vi "aal_Complex Modulator(complex input).vi"(1 "reset ?":bool, 2 "fs":dbl=1024.0 min=-0.5 max=0.5 format="%.2f", 3 "frequency":dbl min=-0.5 max=0.5 format="%.2f", 4 "x":cdb[](array[numeric])) -> (0 "y":cdb[](array[numeric]))   [LabVIEW 2017, in "NI_AALPro.lvlib"]
doc: "Modulates the signal to frequency. The center frequency should be normalized (-0.5, 0.5)."
uses:
  NI_AALPro.lvlib
  <resource>/lvanlys.dll
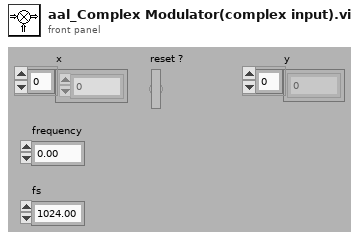
[diagram p1: front panel]
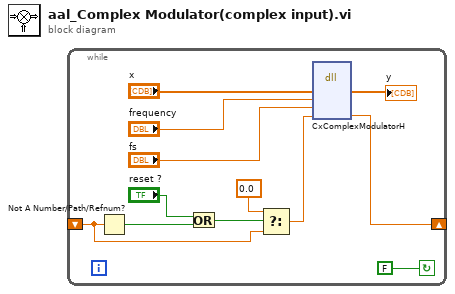
[diagram p0: block diagram]
diagram:
  n1 = while {
    shift-left: _ -> [w11]
    shift-right: [w6] -> _
    stop <- FALSE continue-if-true
    n2 = Not A Number/Path/Refnum?(number/path/refnum=w11) -> (NaN/Path/Refnum?=w2:bool)
    n3 = Or(x="reset ?", y=w2) -> (x .or. y?=w5:bool)
    n4 = Select(t=0.0, s=w5, f=w11) -> (s? t:f=w7:dbl)
    n5 = dll-call lib="C:/Program Files (x86)/National Instruments/LabVIEW 2017/resource/lvanlys.*" fn="CxComplexModulatorH"("x"="x", "fc"="frequency", "fs"="fs", "initial_phase"=w7) -> ("x"=→"y":cdb[], "initial_phase"=w6:dbl)  [unwired: 6 in, 2 out]
  }
